vi "Server Create Command Event.vi"(8 "error in":errorcluster, 11 "server ref":refnum<vi>) -> (0 "error out":errorcluster, 3 "server command event":refnum<user-event>)   [LabVIEW 2013]
doc: "Create user event for server operation commands. I.e.: for events generated by server and processed by TWM."
uses:
  Server Event.ctl
  Server Client Request.ctl
  Server Event Command.ctl
  Server Session Reference.ctl
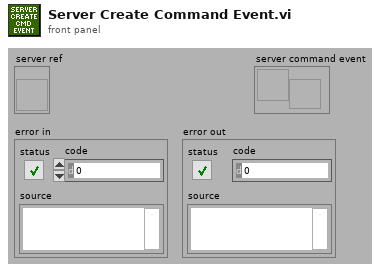
[diagram p1: front panel]
types:
  T1 = typedef "Server Session Reference.ctl" = refnum<vi>
  T2 = typedef "Server Event.ctl" = cluster{"client request":T3, "command":T4}
  T3 = typedef "Server Client Request.ctl" = cluster{"info data":string, "answer handle":i32}
  T4 = typedef "Server Event Command.ctl" = enum16{"None", "Restart", "Identify", "Set measurement", "Start", "Get status", "Get result", "Stop", "Set corrections", "Get algorithm info"}
  T5 = typedef "Server Session.ctl" = cluster{"cmd event":variant, "answer event":variant}
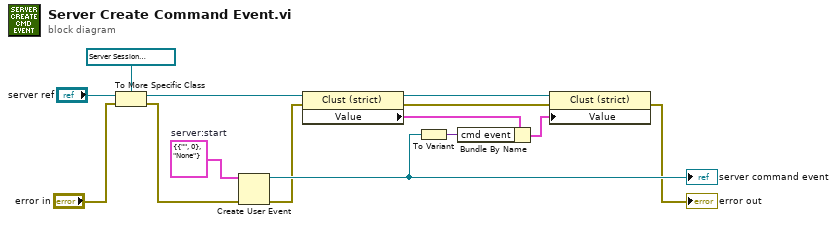
[diagram p0: block diagram]
diagram:
  w14 = T2 {"client request"={"info data"="", "answer handle"=0}, "command"=enum."None"}  # server:start
  n1 = To More Specific Class(target class=T1 refnum ("server ref"), reference="server ref", error in="error in") -> (specific class reference=w7:T1, error out=w9:errorcluster)
  n2 = Create User Event(user event datatype=w14, error in=w9) -> (user event=w13:refnum<user-event>, error out=w5:errorcluster)
  "server command event" <- w13
  n3 = property class="Clust (strict)"(reference=w7, error in=w5) -> (reference out=w6:T1, error out=w4:errorcluster, "Value"=w3:T5)
  n4 = To Variant(anything=w13) -> (Variant=w1:variant)
  n5 = Bundle By Name(cluster=w3, "cmd event"=w1) -> (w2:T5)
  n6 = property class="Clust (strict)"(reference=w6, error in=w4, "Value"=w2) -> (error out=→"error out":errorcluster)  [unwired: 1 out]
